vi "Plot TopArray ValueChange.vi"(8 "error in (no error)":errorcluster, 9 "OldVal":T1[](array[typedef]), 10 "NewVal":T1[](array[typedef]), 11 "Refs":T2) -> (0 "error out":errorcluster)   [LabVIEW 2021, in "RocketPlot.lvlib"]
uses:
  RocketPlot.lvlib
  TypeDefs/Plot UI references.ctl
  Classes/RocketPlotHandle/RocketPlotHandle.lvclass
  <userlib>/bjustice/TipStripOOPanel/Classes/TipPanelHandle/TipPanelHandle.lvclass
  TypeDefs/Plot top row.ctl
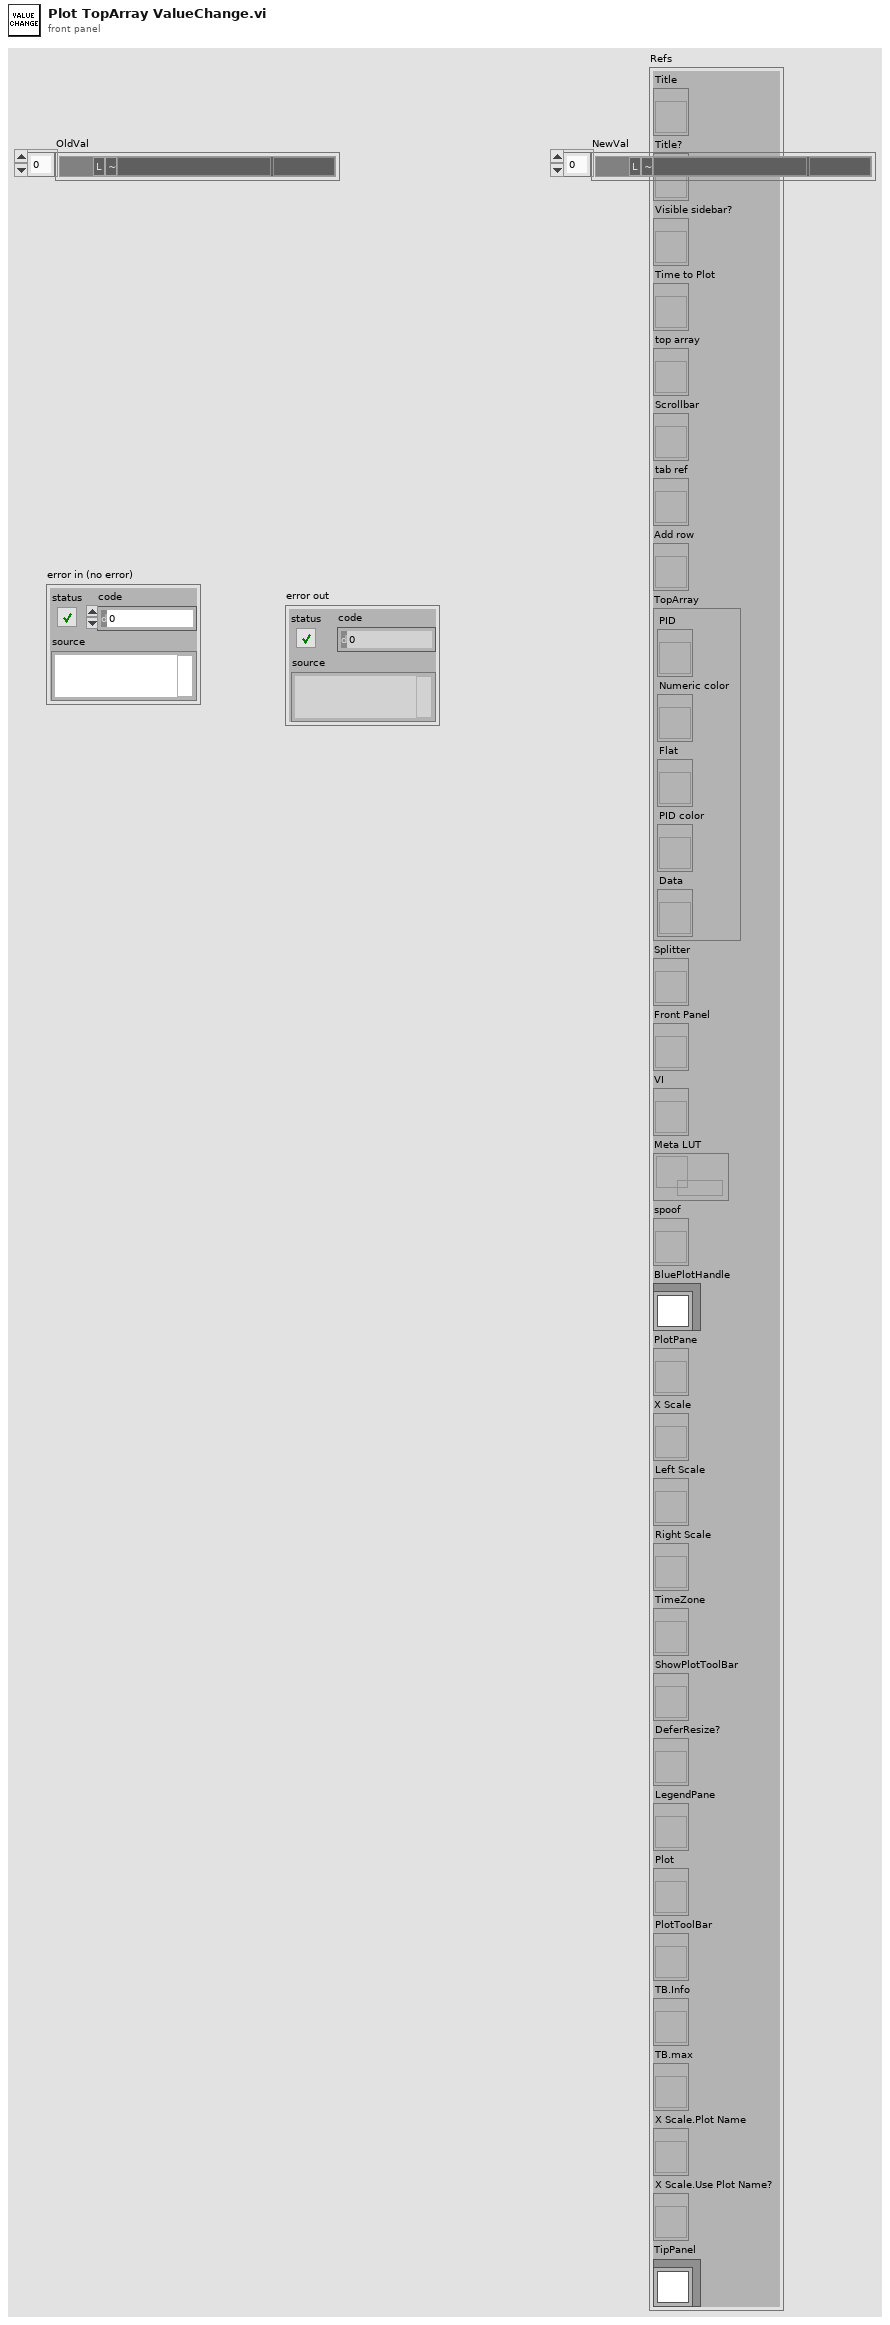
[diagram p1: front panel]
types:
  T1 = typedef "RocketPlot.lvlib/Plot top row.ctl" = cluster{"PID":string, "index":i32, "PID color":u32, "right axis?":bool, "Flatline?":bool, "Numeric color":u32, "Data":string, "Flat":string}
  T2 = typedef "RocketPlot.lvlib/Plot UI references.ctl" = cluster{"Title":refnum<vi>, "Title?":refnum<vi>, "Visible sidebar?":refnum<vi>, "Time to Plot":refnum<vi>, "top array":refnum<vi>, "Scrollbar":refnum<vi>, "tab ref":refnum<vi>, "Add row":refnum<vi>, "TopArray":cluster{"PID":refnum<vi>, "Numeric color":refnum<vi>, "Flat":refnum<vi>, "PID color":refnum<vi>, "Data":refnum<vi>}, "Splitter":refnum<vi>, "Front Panel":refnum<vi>, "VI":refnum<vi>, "Meta LUT":refnum<data-value>, "spoof":refnum<vi>, "BluePlotHandle":refnum<class "RocketPlotHandle.lvclass">, "PlotPane":refnum<vi>, "X Scale":refnum<vi>, "Left Scale":refnum<vi>, "Right Scale":refnum<vi>, "TimeZone":refnum<vi>, "ShowPlotToolBar":refnum<vi>, "DeferResize?":refnum<vi>, "LegendPane":refnum<vi>, "Plot":refnum<vi>, "PlotToolBar":refnum<vi>, "TB.Info":refnum<vi>, "TB.max":refnum<vi>, "X Scale.Plot Name":refnum<vi>, "X Scale.Use Plot Name?":refnum<vi>, "TipPanel":refnum<class "TipPanelHandle.lvclass">}
  T3 = cluster{"PID":bool, "index":bool, "PID color":bool, "right axis?":bool, "Flatline?":bool, "Numeric color":bool, "Data":bool, "Flat":bool}[]
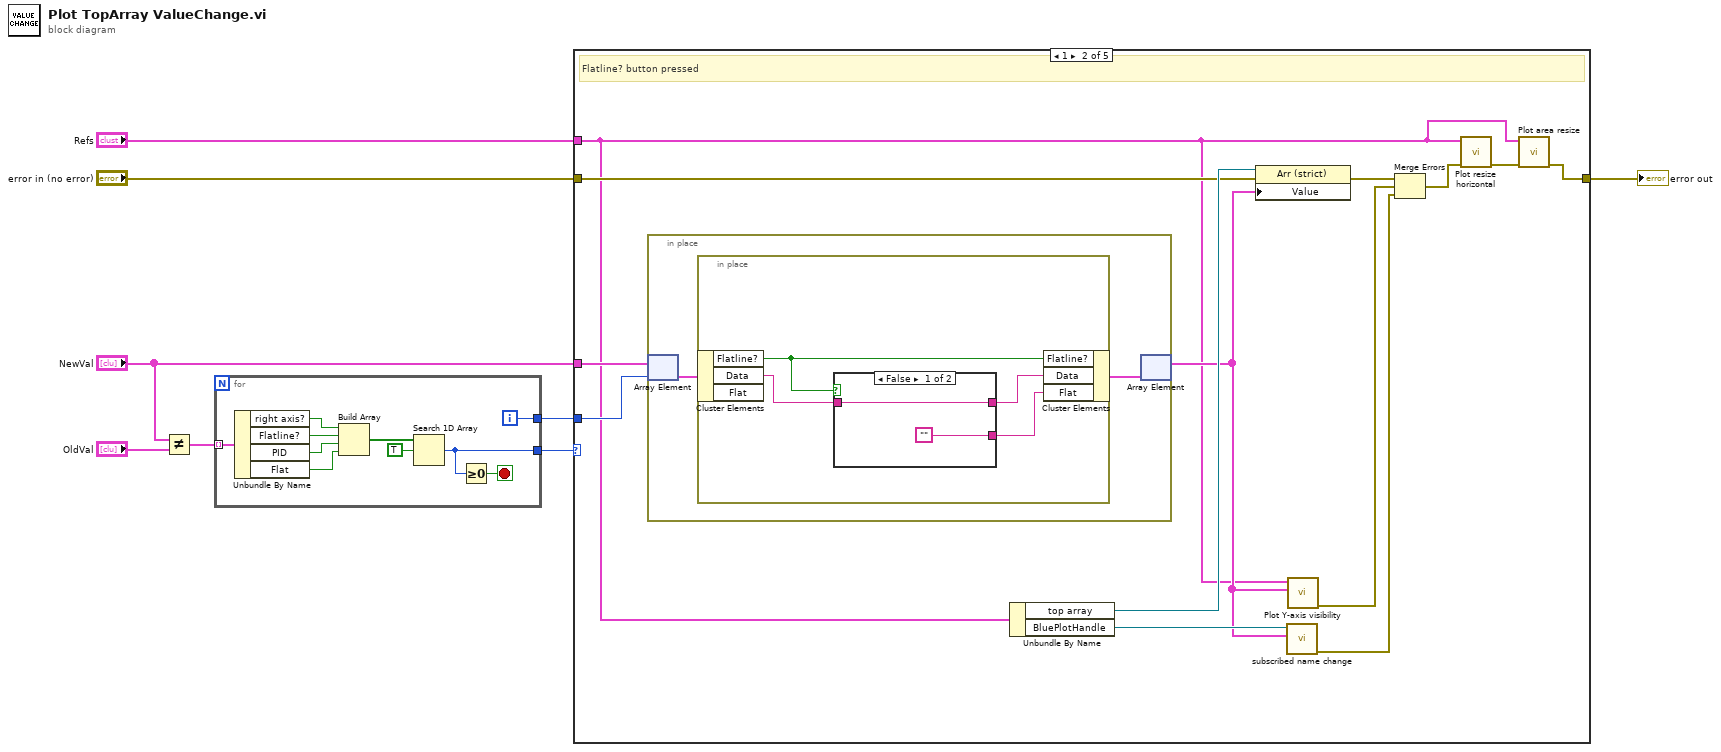
[diagram p0: block diagram]
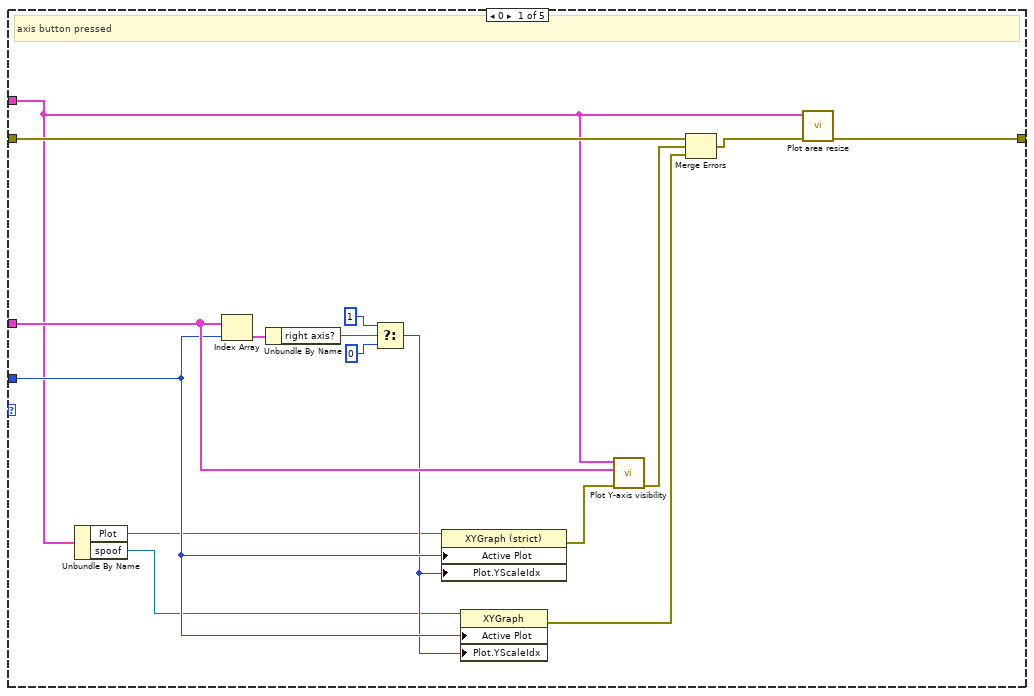
[diagram p2: hidden frame]
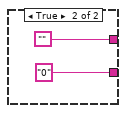
[diagram p3: hidden frame]
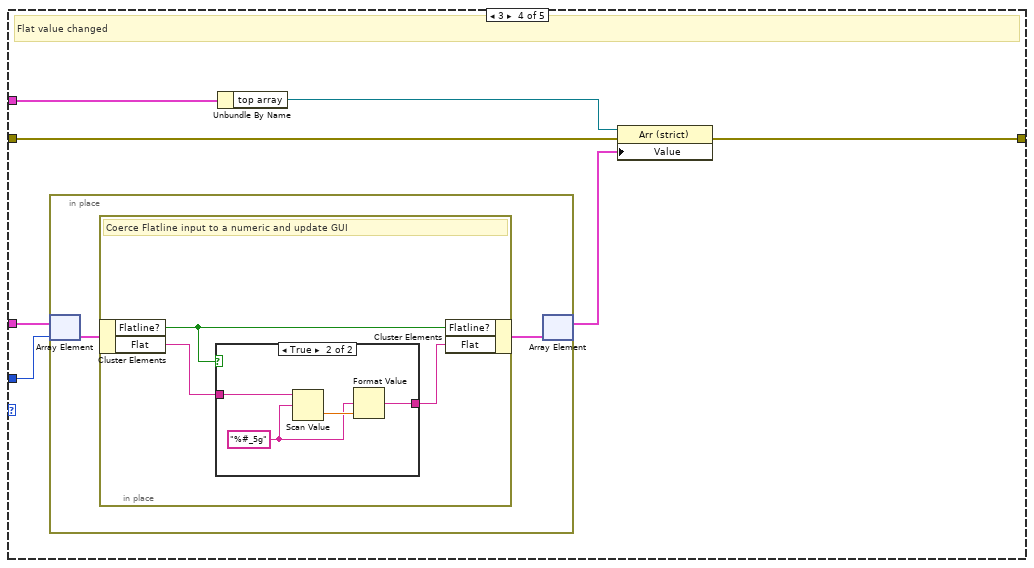
[diagram p5: hidden frame]
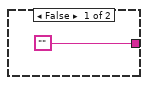
[diagram p6: hidden frame]
diagram:
  n1 = Not Equal?(x="NewVal", y="OldVal") -> (x != y?=w8:T3)
  n2 = for {
    tunnel: w8 -> [w18] mode=indexing
    tunnel: [w12] -> w7
    tunnel: [w11] -> w4
    i -> [w11]
    stop <- w13 stop-if-true
    n3 = Unbundle By Name(w18) -> ("right axis?"=w16:bool, "Flatline?"=w14:bool, "PID"=w10:bool, "Flat"=w9:bool)
    n4 = Build Array(w16, w14, w10, w9) -> (w17:bool[])
    n5 = Search 1D Array(1D array=w17, element=TRUE) -> (index of element=w12:i32)  [unwired: 1 in]
    n6 = Greater Or Equal To 0?(x=w12) -> (x >= 0?=w13:bool)
  }
  n7 = case shown="1" w7 {
    tunnel: "error in (no error)" -> [w26 w42 w58 w63 w76]
    tunnel: [w20 w36 w58 w60 w76] -> w5
    tunnel: w4 -> [w28 w46 _ w59 _]
    tunnel: "NewVal" -> [w29 w47 _ w65 _]
    tunnel: "Refs" -> [w19 w35 _ w64 _]
    frame 0 {
      # "axis button pressed"
      n8 = Unbundle By Name(w19) -> ("Plot"=w23:refnum<vi>, "spoof"=w22:refnum<vi>)
      n9 = Index Array(array=w29, index=w28) -> (element=w34:T1)
      n10 = Unbundle By Name(w34) -> ("right axis?"=w33:bool)
      n11 = Select(t=u32 1 ("Plot.Y Scale Index"), s=w33, f=u32 0 ("Plot.Y Scale Index")) -> (s? t:f=w27:u32)
      n12 = property class="XYGraph (strict)"(reference=w23, "Active Plot"=w28, "Plot.YScaleIdx"=w27) -> (error out=w30:errorcluster)  [unwired: 1 in, 1 out]
      n13 = property class="XYGraph"(reference=w22, "Active Plot"=w28, "Plot.YScaleIdx"=w27) -> (error out=w24:errorcluster)  [unwired: 1 in, 1 out]
      n14 = call "Plot Y-axis visibility.vi"("error in (no error)"=w30, "top array"=w29, "Refs"=w19) -> ("error out"=w25:errorcluster)  [unwired: 8 in]
      n15 = Merge Errors(w26, w25, w24) -> (w21:errorcluster)
      n16 = call "Plot area resize.vi"("error in (no error)"=w21, "Refs"=w19) -> ("error out"=w20:errorcluster)  [unwired: 9 in]
    }
    frame 1 {
      # "Flatline? button pressed"
      n17 = in-place {
        n18 = in-place-array #1(w47, w46) -> (w49:T1)
        n19 = in-place {
          n20 = in-place-cluster #2(w49) -> ("Flatline?"=w53:bool, "Data"=w50:string)  [unwired: 1 out]
          n21 = case shown="False" w53 {
            tunnel: [w54 ""] -> w52
            tunnel: ["" "0"] -> w51
            tunnel: w50 -> [w54 _]
            frame False {
            }
            frame True {
            }
          }
          n22 = in-place-cluster #2("Flatline?"=w53, "Data"=w52, "Flat"=w51) -> (w48:T1)
        }
        n23 = in-place-array #1(w48) -> (w39:T1[])  [unwired: 1 out]
      }
      n24 = Unbundle By Name(w35) -> ("top array"=w43:refnum<vi>, "BluePlotHandle"=w40:refnum<class "RocketPlotHandle.lvclass">)
      n25 = property class="Arr (strict)"(reference=w43, error in=w42, "Value"=w39) -> (error out=w41:errorcluster)  [unwired: 1 out]
      n26 = call "subscribed name change.vi"("top array"=w39, "BluePlotHandle"=w40) -> ("error out"=w38:errorcluster)  [unwired: 9 in]
      n27 = call "Plot Y-axis visibility.vi"("top array"=w39, "Refs"=w35) -> ("error out"=w45:errorcluster)  [unwired: 9 in]
      n28 = Merge Errors(w41, w45, w38) -> (w44:errorcluster)
      n29 = call "Plot resize horizontal.vi"("error in (no error)"=w44, "Refs"=w35) -> ("error out"=w37:errorcluster)  [unwired: 9 in]
      n30 = call "Plot area resize.vi"("error in (no error)"=w37, "Refs"=w35) -> ("error out"=w36:errorcluster)  [unwired: 9 in]
    }
    frame 2 {
      # "PID string changed"
    }
    frame 3 {
      # "Flat value changed"
      n31 = in-place {
        n32 = in-place-array #3(w65, w59) -> (w67:T1)
        n33 = in-place {
          # "Coerce Flatline input to a numeric and update GUI"
          n34 = in-place-cluster #4(w67) -> ("Flatline?"=w70:bool, "Flat"=w68:string)
          n35 = case shown="True" w70 {
            tunnel: ["" w72] -> w69
            tunnel: w68 -> [_ w75]
            frame False {
            }
            frame True {
              w73 = "%#_5g"
              n36 = Scan Value(string=w75, format string=w73) -> (value=w74:dbl)  [unwired: 1 in, 1 out]
              n37 = Format Value(format string=w73, value (0)=w74) -> (output string=w72:string)  [unwired: 1 in]
            }
          }
          n38 = in-place-cluster #4("Flatline?"=w70, "Flat"=w69) -> (w66:T1)
        }
        n39 = in-place-array #3(w66) -> (w62:T1[])  [unwired: 1 out]
      }
      n40 = Unbundle By Name(w64) -> ("top array"=w61:refnum<vi>)
      n41 = property class="Arr (strict)"(reference=w61, error in=w63, "Value"=w62) -> (error out=w60:errorcluster)  [unwired: 1 out]
    }
    frame -1, Default {
      # "do nothing"
    }
  }
  "error out" <- w5
